vi "Velocity_FFT.vi"(6 "Freq_Cutoff":dbl, 7 "Samples":i32, 9 "Sampling Frequency":dbl) -> (0 "error out":errorcluster, 1 "Frequency":dbl, 2 "t_vect":dbl[](array[numeric]), 3 "Peaks":dbl[][](array[numeric]), 4 "XY Graph":cluster{"Y":dbl[], "Y":dbl[]}[](graph), 5 "XY Graph 2":cluster{"Y":dbl[], "Y":dbl[]}[](graph))   [LabVIEW 2018]
panel:
  out "Phase":dbl[](array[numeric])
  out "Magnitude":dbl[](array[numeric])
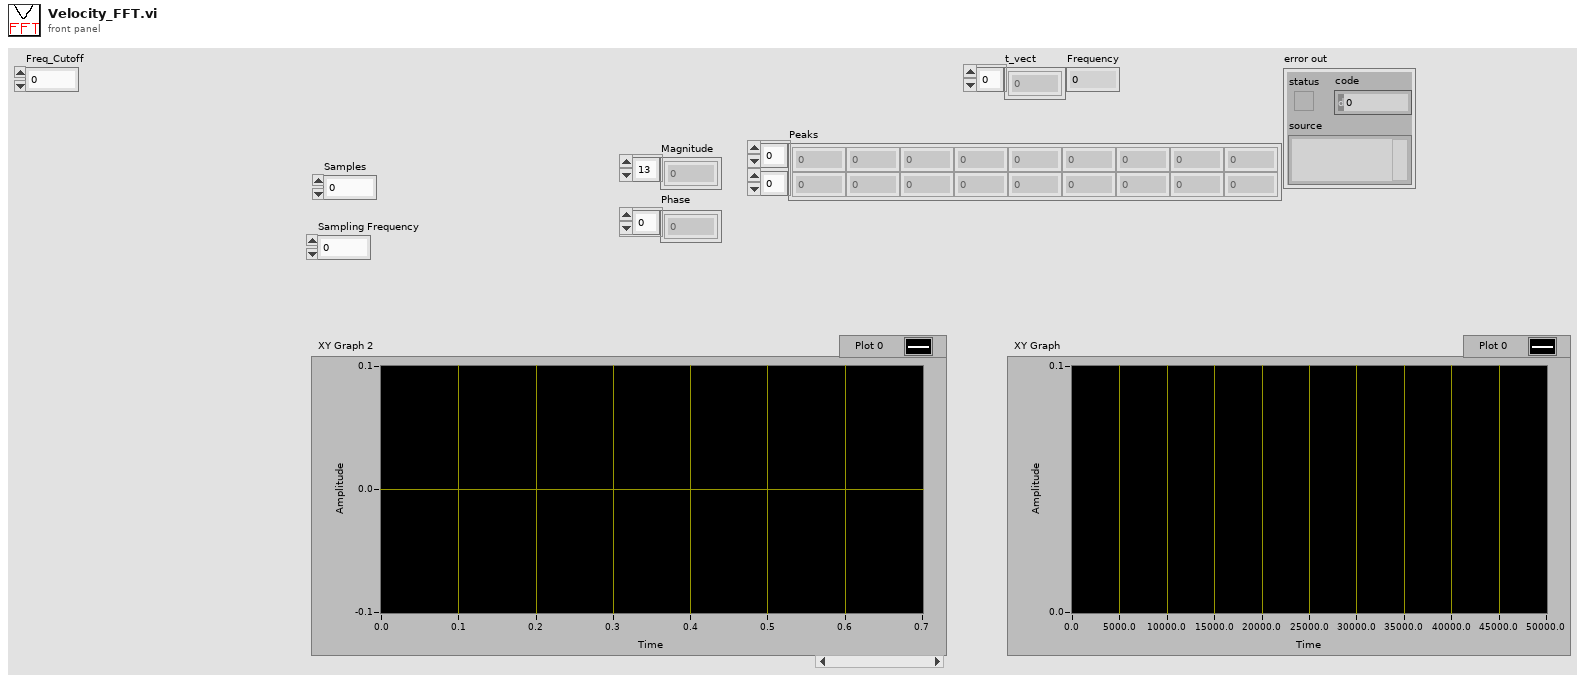
[diagram p1: front panel]
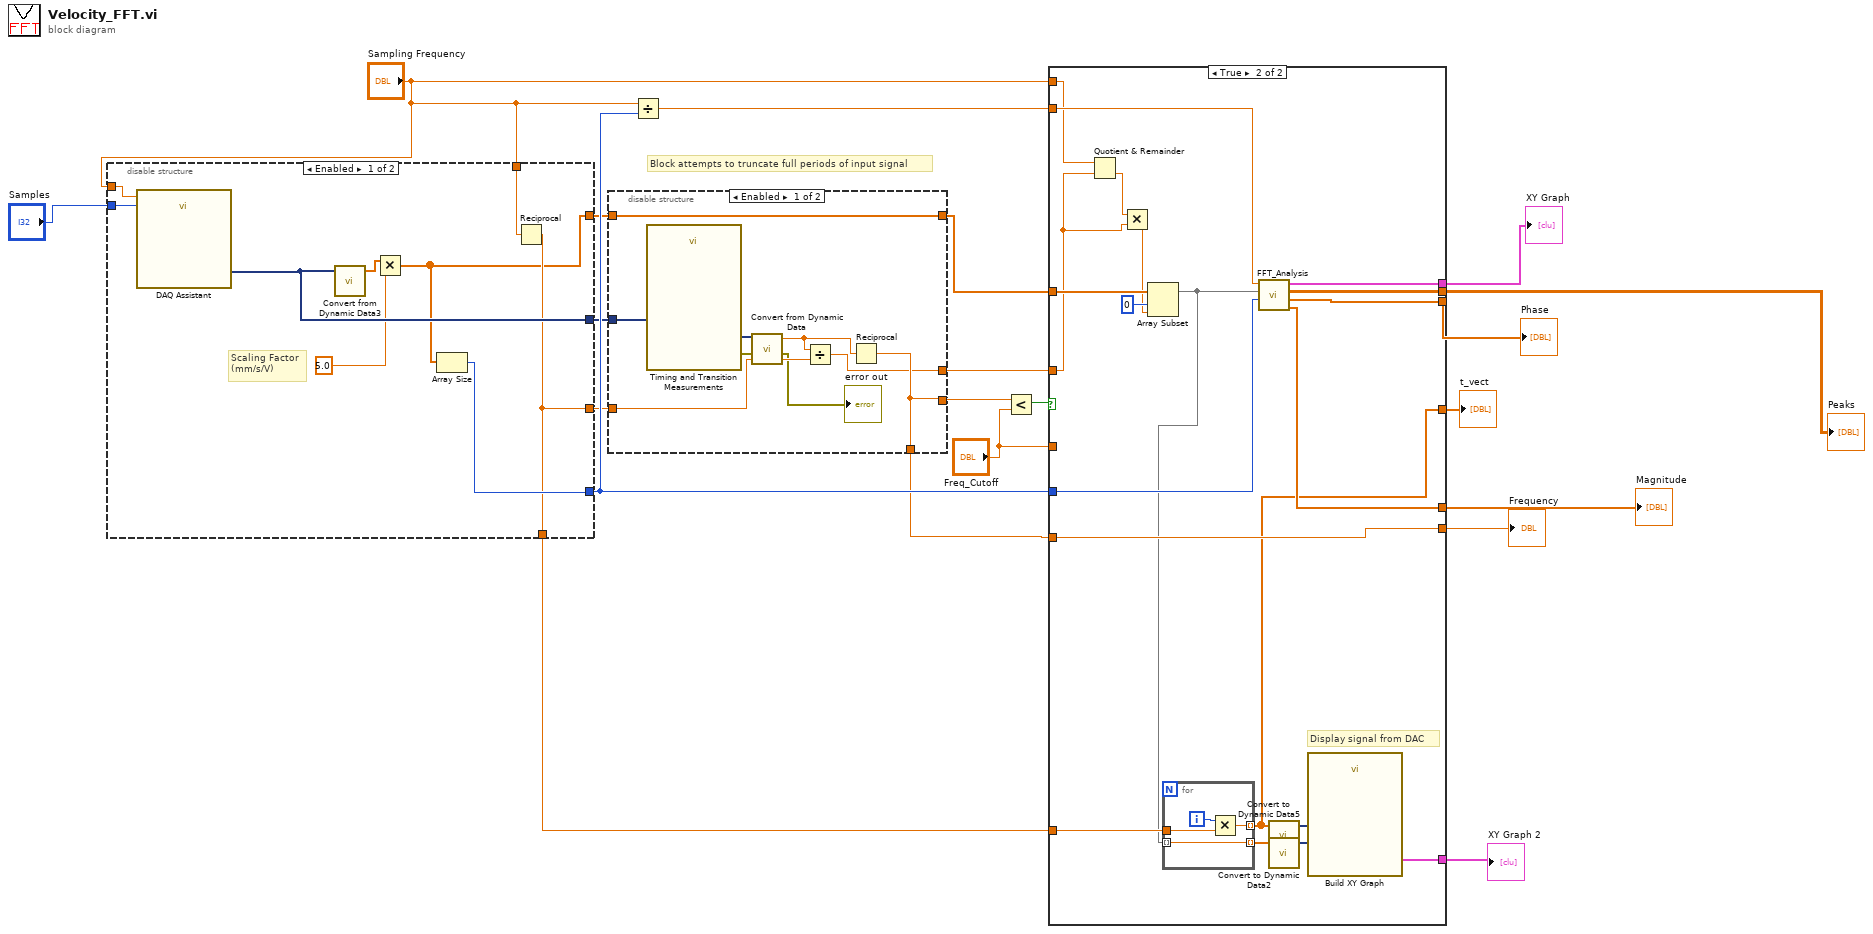
[diagram p0: block diagram]
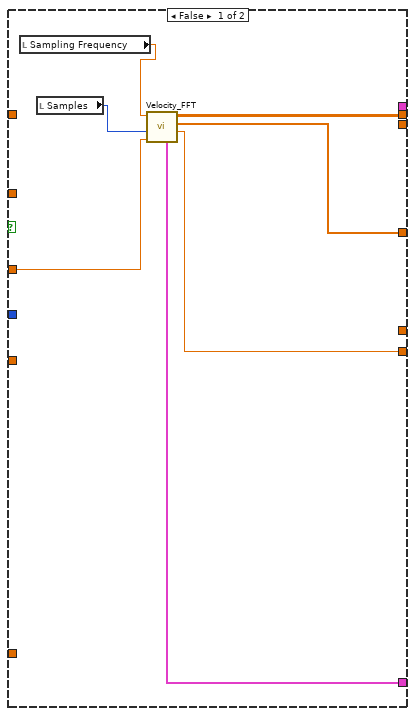
[diagram p2: hidden frame]
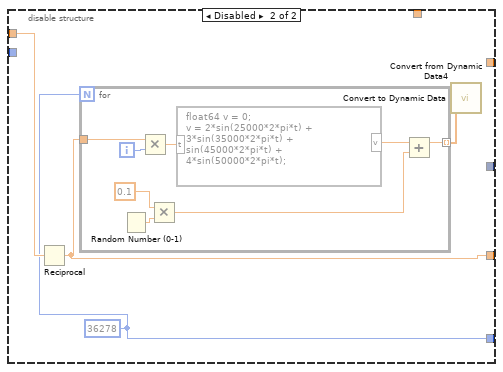
[diagram p4: hidden frame]
diagram:
  # "Block attempts to truncate full periods of input signal"
  n1 = disable-structure shown="Enabled" {
    disable-tunnel: "Sampling Frequency" -> [w29 w35]
    disable-tunnel: [w26 w34] -> w17
    disable-tunnel: [w30 w32] -> w20
    disable-tunnel: "Sampling Frequency" -> [w28 _]
    disable-tunnel: [w27 _] -> w19
    disable-tunnel: [w24 _] -> w16
    disable-tunnel: [w26 _] -> w5
    disable-tunnel: "Samples" -> [w25 _]
    frame Enabled {
      # "Scaling Factor\n(mm/s/V)"
      n2 = call "DAQ Assistant"("rate"=w29, "number of samples"=w25) -> ("data"=w27:dynamicdata)  [unwired: 15 in, 2 out]
      n3 = call "Convert from Dynamic Data3"("Dynamic Data Type"=w27) -> ("Array"=w23:dbl[])  [unwired: 3 in]
      n4 = Multiply(x=w23, y=5.0) -> (x*y=w24:dbl[])
      n5 = Array Size(array=w24) -> (size(s)=w30:i32)
      n6 = Reciprocal(x=w28) -> (1/x=w26:dbl)
    }
    frame Disabled {
      w32 = 36278 ("Samples")
      n7 = Reciprocal(x=w35) -> (1/x=w34:dbl)
      n8 = for {
        N: w32 -> [_]
        tunnel: w34 -> [w43]
        tunnel: [w37] -> w33 mode=indexing
        i -> [w40]
        n9 = Random Number (0-1)() -> (number: 0 to 1=w38:dbl)
        n10 = Multiply(x=w43, y=w40) -> (x*y=w42:dbl)
        n11 = Multiply(x=0.1, y=w38) -> (x*y=w36:dbl)
        n12 = formula code="float64 v = 0;\nv = 2*sin(25000*2*pi*t) +\n3*sin(35000*2*pi*t) +\nsin(45000*2*pi*t) +\n4*sin(50000*2*pi*t);"("t"=w42) -> ("v"=w41:dbl)
        n13 = Add(x=w41, y=w36) -> (x+y=w37:dbl)
      }
      n14 = call "Convert to Dynamic Data"("Array"=w33) -> ("Dynamic Data Type"=w31:dynamicdata)  [unwired: 3 in]
      n15 = call "Convert from Dynamic Data4"("Dynamic Data Type"=w31) -> ()  [unwired: 3 in, 1 out]
    }
  }
  n16 = disable-structure shown="Enabled" {
    disable-tunnel: w19 -> [w49 _]
    disable-tunnel: w17 -> [w48 _]
    disable-tunnel: [w45 w52] -> w15
    disable-tunnel: w16 -> [w45 w52]
    disable-tunnel: [w46 _] -> w8
    disable-tunnel: [w46 _] -> w9
    disable-tunnel: [w44 _] -> w3
    frame Enabled {
      n17 = call "Timing and Transition Measurements"("Signals"=w49) -> ("error out"=→"error out":errorcluster, "Period"=w51:dynamicdata)  [unwired: 9 in]
      n18 = call "Convert from Dynamic Data"("Dynamic Data Type"=w51) -> ("Scalar"=w50:dbl)  [unwired: 3 in]
      n19 = Divide(x=w50, y=w48) -> (x/y=w44:dbl)
      n20 = Reciprocal(x=w50) -> (1/x=w46:dbl)
    }
    frame Disabled {
    }
  }
  n21 = Divide(x="Sampling Frequency", y=w20) -> (x/y=w21:dbl)
  n22 = Less?(x=w9, y="Freq_Cutoff") -> (x < y?=w10:bool)
  n23 = case shown="True" w10 {
    tunnel: w21 -> [_ w65]
    tunnel: w20 -> [_ w79]
    tunnel: w15 -> [_ w70]
    tunnel: [_ w78] -> w14
    tunnel: [w57 w77] -> w13
    tunnel: [_ w76] -> w12
    tunnel: [_ w75] -> w11
    tunnel: w8 -> [_ w74]
    tunnel: [w56 w74] -> w7
    tunnel: [w55 w68] -> w6
    tunnel: w5 -> [_ w69]
    tunnel: [w53 w67] -> w4
    tunnel: w3 -> [_ w60]
    tunnel: "Sampling Frequency" -> [_ w62]
    tunnel: "Freq_Cutoff" -> [w54 _]
    frame False {
      n24 = local read "Sampling Frequency"() -> (w58:dbl)
      n25 = local read "Samples"() -> (w59:i32)
      n26 = call "Velocity_FFT.vi"("Freq_Cutoff"=w54, "Samples"=w59, "Sampling Frequency"=w58) -> ("Frequency"=w56:dbl, "t_vect"=w55:dbl[], "Peaks"=w57:dbl[][], "XY Graph"=w53:cluster{"Y":dbl[], "Y":dbl[]}[])  [unwired: 1 in, 2 out]
    }
    frame True {
      # "Display signal from DAC"
      n27 = Quotient & Remainder(x=w62, y=w60) -> (floor(x/y)=w64:dbl)  [unwired: 1 out]
      n28 = Multiply(x=w64, y=w60) -> (x*y=w61:dbl)
      n29 = Array Subset(array=w70, index=0, length=w61) -> (w63:dbl[])
      n30 = for {
        tunnel: w63 -> [w83] mode=indexing
        tunnel: [w83] -> w72 mode=indexing
        tunnel: w69 -> [w81]
        tunnel: [w80] -> w68 mode=indexing
        i -> [w82]
        n31 = Multiply(x=w82, y=w81) -> (x*y=w80:dbl)
      }
      n32 = call "FFT_Analysis.vi"("Length of Sample"=w79, "Data"=w63, "T_vect"=w65) -> ("Magnitude"=w75:dbl[], "Phase"=w76:dbl[], "Peaks"=w77:dbl[][], "XY Graph"=w78:cluster{"Y":dbl[], "Y":dbl[]}[])  [unwired: 4 in]
      n33 = call "Convert to Dynamic Data5"("Array"=w68) -> ("Dynamic Data Type"=w73:dynamicdata)  [unwired: 3 in]
      n34 = call "Convert to Dynamic Data2"("Array"=w72) -> ("Dynamic Data Type"=w71:dynamicdata)  [unwired: 3 in]
      n35 = call "Build XY Graph"("Y Input"=w71, "X Input"=w73) -> ("XY Graph"=w67:cluster{"X":dbl[], "Y":dbl[]}[])  [unwired: 8 in, 1 out]
    }
  }
  "Phase" <- w12
  "XY Graph" <- w14
  "Peaks" <- w13
  "t_vect" <- w6
  "Frequency" <- w7
  "Magnitude" <- w11
  "XY Graph 2" <- w4
